vi "Insert Normal Controls to [5,5] Array.vi"(7 "controls":refnum<vi>[](array[refnum]), 9 "2-D controls references":refnum<vi>[][](array[refnum])) -> (1 "2-D controls references out":refnum<vi>[][](array[refnum]), 3 "controls out":refnum<vi>[](array[refnum]))   [LabVIEW 2018, in "NISAST VI Scripting.lvlib" / "VI.lvlib" / "Front Panel.lvlib"]
uses:
  Front Panel.lvlib
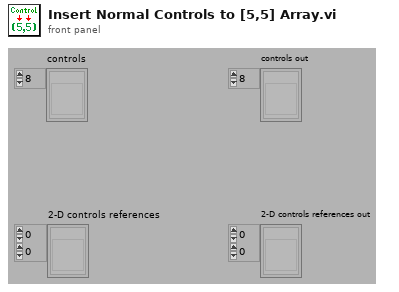
[diagram p1: front panel]
types:
  T1 = cluster{"Index (row)":i32, "Disabled Index (col)":i32}[]
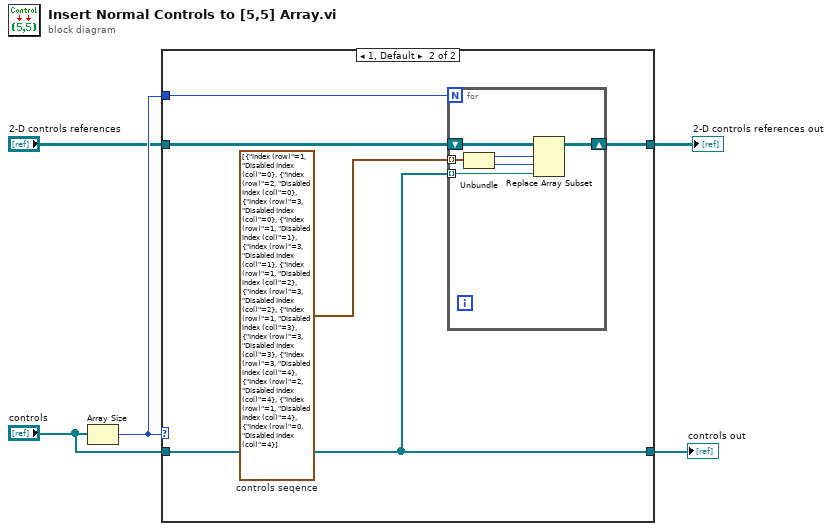
[diagram p0: block diagram]
diagram:
  n1 = Array Size(array="controls") -> (size(s)=w3:i32)
  n2 = case shown="1, Default" w3 {
    tunnel: "2-D controls references" -> [w7 w11]
    tunnel: [w7 w9] -> w5
    tunnel: "controls" -> [w6 w8]
    tunnel: w3 -> [_ w12]
    tunnel: [w6 w8] -> w1
    frame 0 {
    }
    frame 1, Default {
      w10 = T1 [{"Index (row)"=1, "Disabled Index (col)"=0}, {"Index (row)"=2, "Disabled Index (col)"=0}, {"Index (row)"=3, "Disabled Index (col)"=0}, {"Index (row)"=1, "Disabled Index (col)"=1}, {"Index (row)"=3, "Disabled Index (col)"=1}, {"Index (row)"=1, "Disabled Index (col)"=2}, {"Index (row)"=3, "Disabled Index (col)"=2}, {"Index (row)"=1, "Disabled Index (col)"=3}, {"Index (row)"=3, "Disabled Index (col)"=3}, {"Index (row)"=3, "Disabled Index (col)"=4}, {"Index (row)"=2, "Disabled Index (col)"=4}, {"Index (row)"=1, "Disabled Index (col)"=4}, {"Index (row)"=0, "Disabled Index (col)"=4}]  # controls seqence
      n3 = for {
        N: w12 -> [_]
        tunnel: w8 -> [w13] mode=indexing
        shift-right: [w17] -> w9
        shift-left: w11 -> [w18]
        tunnel: w10 -> [w16] mode=indexing
        n4 = Unbundle(w16) -> ("Index (row)"=w15:i32, "Disabled Index (col)"=w14:i32)
        n5 = Replace Array Subset(array=w18, new element=w13, index (row)=w15, index (col)=w14) -> (w17:refnum<vi>[][])
      }
    }
  }
  "2-D controls references out" <- w5
  "controls out" <- w1
